vi "Reflective Tape Processing.vi"() -> ()   [LabVIEW 2014]
uses:
  <vilib>/Rock Robotics/WPI/Camera/WPI_CameraSettings Read MJPG.ctl
  <vilib>/Rock Robotics/WPI/Camera/WPI_CameraImageSize.ctl
  Program Files (x86)/National Instruments/LabVIEW 2014/examples/FRC/roboRIO/Vision/2015 Vision Example/Vision Support Code/Camera Types.ctl
  <vilib>/vision/NI_Vision_Development_Module.lvlib
panel:
  in  "Camera Type":T1=enum."MS HD3000 square"
  in  "Image Path":path=path "Sample Images/KicoffFilmingVision"
  in  "image files":string[](array[string])
  in  "Aspect Fudge Factor":dbl=1.0
  out "Detected Totes":T2(array[cluster]) {"Normalized Rect"."Numeric 5" format="%#_2g"; "Normalized Rect"."Numeric 3" format="%#_2g"; "Normalized Rect"."Numeric 2" format="%#_2g"; "Normalized Rect"."Numeric" format="%#_2g"}
  in  "Score Threshold":dbl=75.0
  in  "Source":enum32{"Files", "Camera"}(tab)
  in  "Images":i32(listbox)
  in  "Folder Location":path=path "Sample Images/KicoffFilmingVision"
  in  "Camera Settings":T3={"fps"=20, "compression"=30, "Image Size"=enum."320x240"}
  in  "Camera Address":string="USB 1"
  in  "Annotate":bool=TRUE
  out "ms to process":u32
  out "Sorted Scores":T5(array[cluster]) {"Aspect Ratio" format="%#_3g"; "Area Score" format="%#_3g"; "X" format="%#_3g"; "Y" format="%#_3g"}
  out "Particles":i32
  in  "Ring Light Color":T6={"Hue"={101.37467765958063, 64.10933859299683}, "Sat"={88.03571428571429, 255.0}, "Val"={133.57142857142858, 255.0}} {"Hue" scale=0.0..255.0 scale format="%#_3g"}
  out "Masked":T7(plugin-control)
  out "Original Image":T7(plugin-control)
  # "Instructions:\nUse Source to select image files from a directory or use a USB or IP camera connected to your laptop.\nUse the Color of a ring light to threshold and build particles. Adjust calibration if needed.\nSmall modifications to the diagram will allow for intensity processing instead of color.\nAnnotations show the rectangle and the scores from top to bottom."
  # "Density Profile"
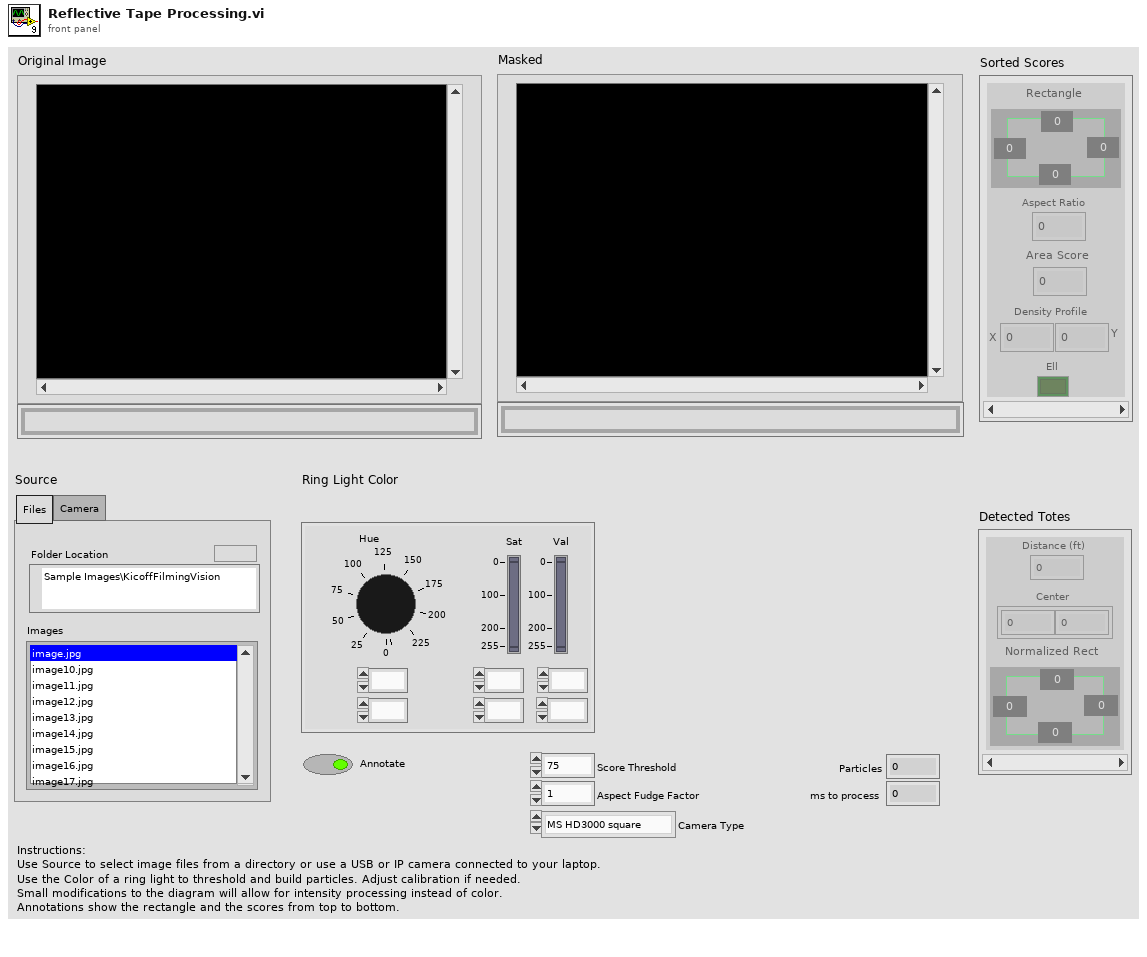
[diagram p1: front panel]
types:
  T1 = typedef "Camera Types.ctl" = enum16{"206", "1011", "1013", "MS HD3000 square", "MS HD3000 640x480"}
  T2 = cluster{"Distance (ft)":dbl, "Center":cluster{dbl, dbl}, "Normalized Rect":cluster{"Numeric":dbl, "Numeric 2":dbl, "Numeric 3":dbl, "Numeric 5":dbl}}[]
  T3 = typedef "WPI_CameraSettings Read MJPG.ctl" = cluster{"fps":i32, "compression":i32, "Image Size":T4}
  T4 = typedef "WPI_CameraImageSize.ctl" = enum16{"640x480", "320x240", "160x120", "Custom"}
  T5 = cluster{"Rectangle":cluster{"Numeric":dbl, "Numeric 2":dbl, "Numeric 3":dbl, "Numeric 5":dbl}, "Aspect Ratio":dbl, "Area Score":dbl, "X":dbl, "Y":dbl, "Ell":bool}[]
  T6 = cluster{"Hue":cluster{dbl, dbl}, "Sat":cluster{dbl, dbl}, "Val":cluster{dbl, dbl}}
  T7 = typedef "IMAQ Image.ctl" = refnum<image>
  T8 = typedef "Image Type" = u32
  T9 = typedef "Particle Parameters" = i32
  T10 = cluster{"Bounding box":cluster{"left":dbl, "top":dbl, "right":dbl, "bottom":dbl}, "Aspect Ratio":dbl, "Area Score":dbl, "X Mask":dbl, "Y Mask":dbl, "Ell":bool}[]
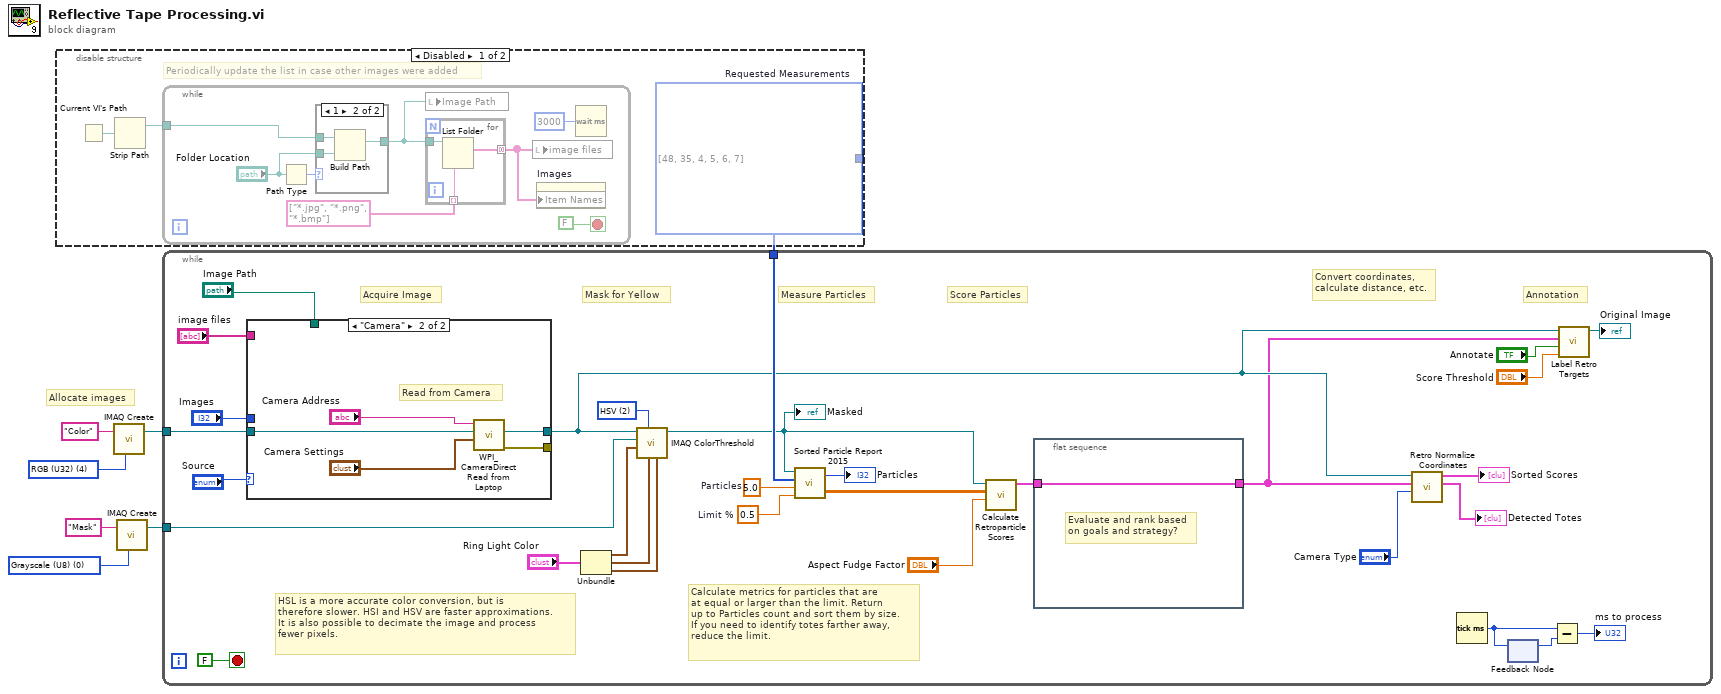
[diagram p0: block diagram]
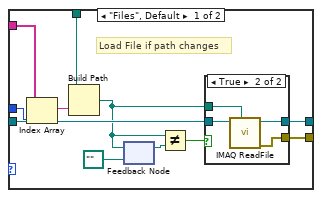
[diagram p4: hidden frame]
diagram:
  w4 = T8 0 items=["Grayscale (U8)", "Grayscale (I16)", "Grayscale (SGL)", "Complex (CSG)", "RGB (U32)", "HSL (U32)", "RGB (U64)", "Grayscale (U16)"] ("Image Type")
  w6 = T8 4 items=["Grayscale (U8)", "Grayscale (I16)", "Grayscale (SGL)", "Complex (CSG)", "RGB (U32)", "HSL (U32)", "RGB (U64)", "Grayscale (U16)"] ("Image Type")
  # "Allocate images"
  n1 = disable-structure shown="Disabled" {
    disable-tunnel: [w10 _] -> w1
    frame Disabled {
      w10 = T9[] [48, 35, 4, 5, 6, 7] items=["Center of Mass X", "Center of Mass Y", "First Pixel X", "First Pixel Y", "Bounding Rect Left", "Bounding Rect Top", "Bounding Rect Right", "Bounding Rect Bottom", "Max Feret Diameter Start X", "Max Feret Diameter Start Y", "Max Feret Diameter End X", "Max Feret Diameter End Y", "Max Horiz. Segment Length Left", "Max Horiz. Segment Length Right", "Max Horiz. Segment Length Row", "-", "Bounding Rect Width", "Bounding Rect Height", "Bounding Rect Diagonal", "Perimeter", "Convex Hull Perimeter", "Holes' Perimeter", "Max Feret Diameter", "Equivalent Ellipse Major Axis", "Equivalent Ellipse Minor Axis", "Equivalent Ellipse Minor Axis (Feret)", "Equivalent Rect Long Side", "Equivalent Rect Short Side", "Equivalent Rect Diagonal", "Equivalent Rect Short Side (Feret)", "Average Horiz. Segment Length", "Average Vert. Segment Length", "Hydraulic Radius", "Waddel Disk Diameter", "-", "Area", "Holes' Area", "Particle & Holes' Area", "Convex Hull Area", "Image Area", "-", "Number of Holes", "Number of Horiz. Segments", "Number of Vert. Segments", "-", "Orientation", "Max Feret Diameter Orientation", "-", "% Area/Image Area", "% Area/(Particle & Holes' Area)", "Ratio of Equivalent Ellipse Axes", "Ratio of Equivalent Rect Sides", "-", "Elongation Factor", "Compactness Factor", "Heywood Circularity Factor", "Type Factor", "-", "Sum X", "Sum Y", "Sum XX", "Sum XY", "Sum YY", "Sum XXX", "Sum XXY", "Sum XYY", "Sum YYY", "-", "Moment of Inertia XX", "Moment of Inertia XY", "Moment of Inertia YY", "Moment of Inertia XXX", "Moment of Inertia XXY", "Moment of Inertia XYY", "Moment of Inertia YYY", "Norm. Moment of Inertia XX", "Norm. Moment of Inertia XY", "Norm. Moment of Inertia YY", "Norm. Moment of Inertia XXX", "Norm. Moment of Inertia XXY", "Norm. Moment of Inertia XYY", "Norm. Moment of Inertia YYY", "Hu Moment 1", "Hu Moment 2", "Hu Moment 3", "Hu Moment 4", "Hu Moment 5", "Hu Moment 6", "Hu Moment 7"]  # Requested Measurements
      # "Periodically update the list in case other images were added"
      n2 = Current VI's Path() -> (path=w9:path)
      n3 = Strip Path(path=w9) -> (stripped path=w8:path)  [unwired: 1 out]
      n4 = while {
        tunnel: w8 -> [w12]
        stop <- FALSE stop-if-true
        n5 = Path Type(1:"Folder Location") -> (0:w14:i16)
        n6 = case shown="1" w14 {
          tunnel: "Folder Location" -> [w19 w22]
          tunnel: [w19 w20] -> w11
          tunnel: w12 -> [_ w21]
          frame 0, Default {
          }
          frame 1 {
            n7 = Build Path(base path=w21, name or relative path=w22) -> (appended path=w20:path)
          }
        }
        n8 = local write "Image Path"(w11) -> ()
        n9 = for {
          tunnel: [w25] -> w15 mode=concatenating
          tunnel: w11 -> [w24]
          tunnel: string[] ["*.jpg", "*.png", "*.bmp"] -> [w23] mode=indexing
          n10 = List Folder(path=w24, pattern=w23) -> (filenames=w25:string[])  [unwired: 2 in, 3 out]
        }
        n11 = local write "image files"(w15) -> ()
        n12 = property on="Images" class="LstBox (strict)"("Item Names"=w15) -> ()  [unwired: 2 in, 2 out]
        n13 = Wait (ms)(milliseconds to wait=u32 3000) -> ()  [unwired: 1 out]
      }
    }
    frame Enabled {
    }
  }
  n14 = call "IMAQ Create"("Image Name"="Color", "Image Type"=w6) -> ("New Image"=w5:T7)  [unwired: 2 in, 2 out]
  n15 = call "IMAQ Create"("Image Name"="Mask", "Image Type"=w4) -> ("New Image"=w2:T7)  [unwired: 2 in, 2 out]
  n16 = while {
    tunnel: w5 -> [w55]
    tunnel: w2 -> [w53]
    tunnel: w1 -> [w47]
    stop <- FALSE stop-if-true
    w44 = 0.5  # Limit %
    w46 = 5.0  # Particles
    w52 = u16 2 items=["RGB", "HSL", "HSV", "HSI"] ("Color Mode")
    # "Calculate metrics for particles that are\nat equal or larger than the limit. Return\nup to Particles count and sort them by size.\nIf you need to identify totes farther away,\nreduce the limit."
    # "Measure Particles"
    # "Convert coordinates,\ncalculate distance, etc."
    # "Annotation"
    # "Score Particles"
    # "Mask for Yellow"
    # "Acquire Image"
    # "HSL is a more accurate color conversion, but is\ntherefore slower. HSI and HSV are faster approximations.\nIt is also possible to decimate the image and process\nfewer pixels."
    n17 = case shown="\"Camera\"" "Source" {
      tunnel: [w67 w78] -> _
      tunnel: [w68 w77] -> w32
      tunnel: w55 -> [w66 w76]
      tunnel: "image files" -> [w58 _]
      tunnel: "Images" -> [w65 _]
      tunnel: "Image Path" -> [w63 _]
      frame "Files", Default {
        # "Load File if path changes"
        n18 = Index Array(array=w58, index=w65) -> (element=w64:string)
        n19 = Build Path(base path=w63, name or relative path=w64) -> (appended path=w59:path)
        n20 = feedback-in #1(w59) -> ()
        n21 = feedback #1(path "" ("appended path")) -> (w61:path)
        n22 = Not Equal?(x=w59, y=w61) -> (x != y?=w62:bool)
        n23 = case shown="True" w62 {
          tunnel: [w69 w73] -> w68
          tunnel: [_ w72] -> w67
          tunnel: w66 -> [w69 w71]
          tunnel: w59 -> [_ w70]
          frame False {
          }
          frame True {
            n24 = call "IMAQ ReadFile"("File Path"=w70, "Image"=w71) -> ("error out"=w72:errorcluster, "Image Out"=w73:T7)  [unwired: 5 in, 3 out]
          }
        }
      }
      frame "Camera" {
        # "Read from Camera"
        n25 = call <vilib>:"WPI_CameraDirect Read from Laptop.vi"("Camera Settings"="Camera Settings", "Image"=w76, "address"="Camera Address") -> ("error out"=w78:errorcluster, "Image Out"=w77:T7)  [unwired: 7 in]
      }
    }
    n26 = Unbundle("Ring Light Color") -> ("Hue"=w51:cluster{dbl, dbl}, "Sat"=w50:cluster{dbl, dbl}, "Val"=w49:cluster{dbl, dbl})
    n27 = call "IMAQ ColorThreshold"("Blue or Luma or Val or Inten Range"=w49, "Green or Sat Range"=w50, "Color Mode"=w52, "Red or Hue Range"=w51, "Image Dst"=w53, "Image Src"=w32) -> ("Image Dst Out"=w37:T7)  [unwired: 4 in, 1 out]
    "Masked" <- w37
    n28 = call "Sorted Particle Report 2015.vi"("Min Area Size %"=w44, "Particle Count Limit"=w46, "Pixel Measurements"=w47, "Image in"=w37) -> ("Sorted Data"=w34:dbl[][], "Particles"=→"Particles":i32)
    n29 = call "Calculate Retroparticle Scores.vi"("Aspect Fudge Factor"="Aspect Fudge Factor", "Sorted Data"=w34, "Image in"=w37) -> ("Scores"=w36:T10)  [unwired: 8 in]
    n30 = flat-sequence {
      tunnel: w36 -> [w57]
      tunnel: [w57] -> w29
      frame #0 {
        # "Evaluate and rank based\non goals and strategy?"
      }
    }
    n31 = call "Retro Normalize Coordinates.vi"("Camera Type"="Camera Type", "Scores"=w29, "Image in"=w32) -> ("Found Totes"=→"Detected Totes":T2, "Sorted Scores"=→"Sorted Scores":T5)  [unwired: 7 in]
    n32 = Tick Count (ms)() -> (millisecond timer value=w42:u32)
    n33 = feedback-in #2(w42) -> ()
    n34 = feedback #2() -> (w43:u32)  [unwired: 1 in]
    n35 = Subtract(x=w42, y=w43) -> (x-y=→"ms to process":u32)
    n36 = call "Label Retro Targets.vi"("Score Threshold"="Score Threshold", "Annotate"="Annotate", "Scores"=w29, "Image in"=w32) -> ("Image out"=→"Original Image":T7)  [unwired: 7 in]
  }
